vi "Element Events.vi"(8 "error in (no error)":errorcluster, 11 "Sequencing Control in":refnum<class "Sequencing Control.lvclass">) -> (0 "error out":errorcluster, 2 "Element Events":refnum<class "Control Event Registrations.lvclass">, 3 "Sequencing Control out":refnum<class "Sequencing Control.lvclass">)   [LabVIEW 2020, in "VolatusSeqGUI.lvlib" / "Sequencing Control.lvclass"]
uses:
  Sequencing Control.lvclass
  C:/dev/lv20CE/relink/lv-volatus/VolatusGUI/GUI Element/GUI Element.lvclass
  C:/dev/lv20CE/relink/lv-volatus/VolatusGUI/OnValueChangeHandler/OnValueChangeHandler.lvclass
  VolatusGUI/Control Event Registrations/Control Event Registrations.lvclass
  VolatusGUI/GUI Element/GUI Element.lvclass/GUI Element.ctl
  Sequencing Control.lvclass/Sequencing Control.ctl
  VolatusGUI/GUI Element/GUI Element.lvclass
  C:/dev/lv20CE/relink/lv-volatus/VolatusSeqGUI/Sequencing Control/Sequencing Control.lvclass
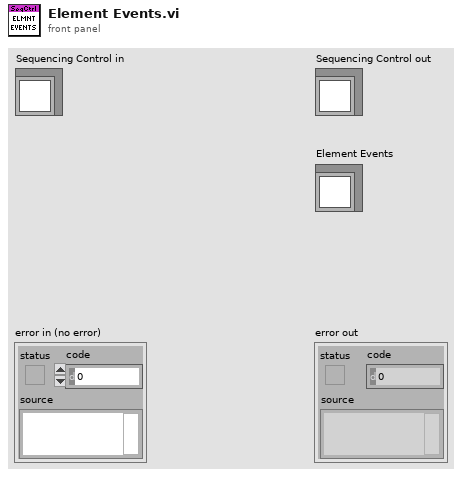
[diagram p1: front panel]
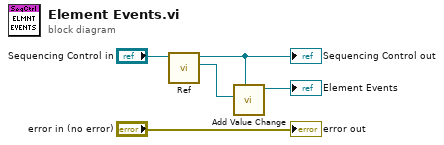
[diagram p0: block diagram]
diagram:
  n1 = call "Ref.vi"("GUI Element in"="Sequencing Control in") -> ("Ref"=w1:refnum<vi>, "GUI Element out"=w2:refnum<class "Sequencing Control.lvclass">)  [unwired: 9 in]
  "Sequencing Control out" <- w2
  n2 = call "Add Value Change.vi"("Control"=w2, "CtlRef"=w1) -> ("Control Event Registrations out"=→"Element Events":refnum<class "Control Event Registrations.lvclass">)  [unwired: 8 in, 1 out]
  "error out" <- "error in (no error)"
